vi "FTW-CodeGen-SelectMenu5.vi"(0 "State In":T2 {"Width" format="%dpx"}, 5 "XRef":refnum<vi>, 7 "Tag":string, 9 "Point":cluster{"H":i32, "V":i32}, 11 "Menu Type":T3(ring)) -> (4 "State Out":T2 {"Width" format="%dpx"}, 6 "Handled?":bool, 8 "Multi Object Popup Options":T1, 10 "Reply":string[](array[string]))   [LabVIEW 2015, in "FTW-Dataflow-Burrow.xnode"]
uses:
  FTW-Dataflow-Burrow.xnode
  FTW-CodeGen-State.ctl
  framework/FTW-CodeGen-XNodeReplyType.ctl
panel:
  # "Inputs"
  # "Outputs"
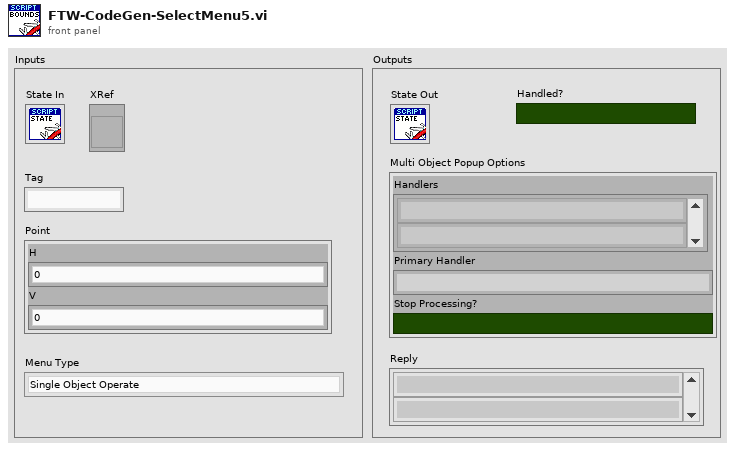
[diagram p1: front panel]
types:
  T1 = cluster{"Handlers":string[], "Primary Handler":string, "Stop Processing?":bool}
  T2 = typedef "FTW-Dataflow-Burrow.xnode/FTW-CodeGen-State.ctl" = cluster{"InputTerminals":cluster{"Wired?":bool, "ID":string, "DataName":string, "DataColor":u32, "Type":variant}[], "EnableTiming?":bool, "Width":i32}
  T3 = enum32{"Single Object Operate", "Single Object Popup", "Multi Object Popup Master", "Multi Object Popup Other"}
  T4 = typedef "FTW-CodeGen-XNodeReplyType.ctl" = enum16{"NoReply", "ForceAdaptToInputs", "UpdateTerms", "GenCode", "GenCode+CosmeticUpdate"}
  T5 = cluster{"Wired?":bool, "ID":string, "DataName":string, "DataColor":u32, "Type":variant}[]
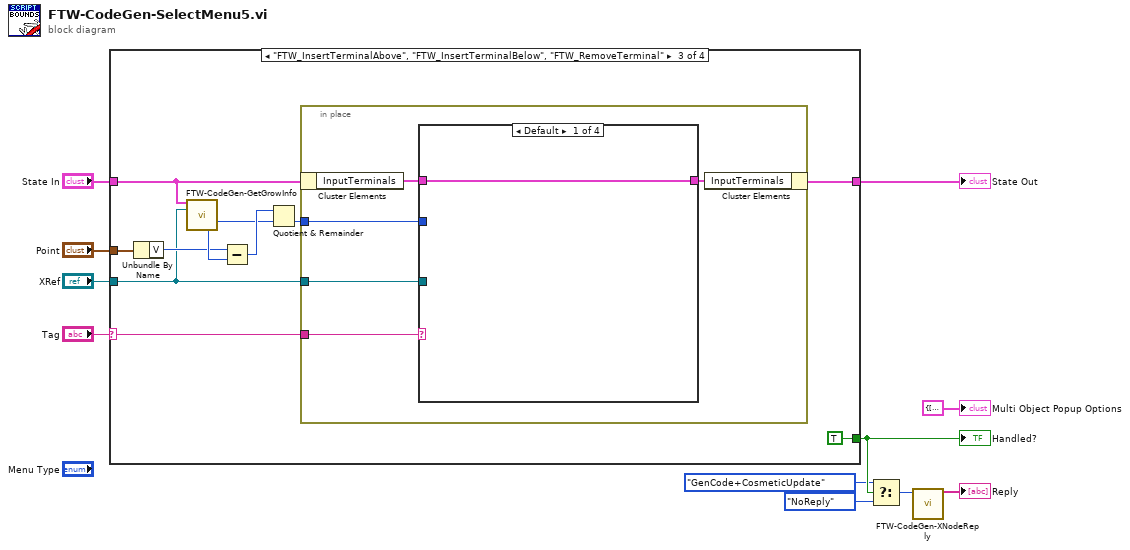
[diagram p0: block diagram]
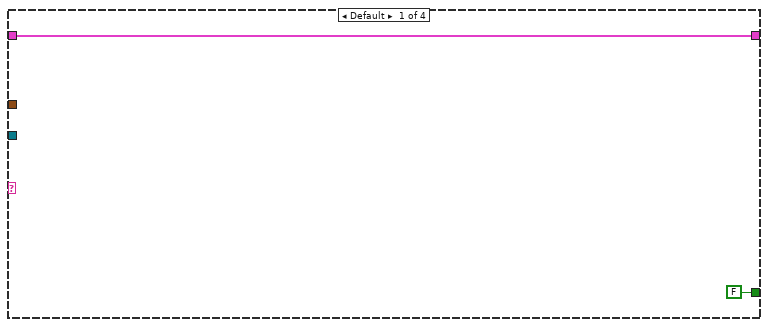
[diagram p2: hidden frame]
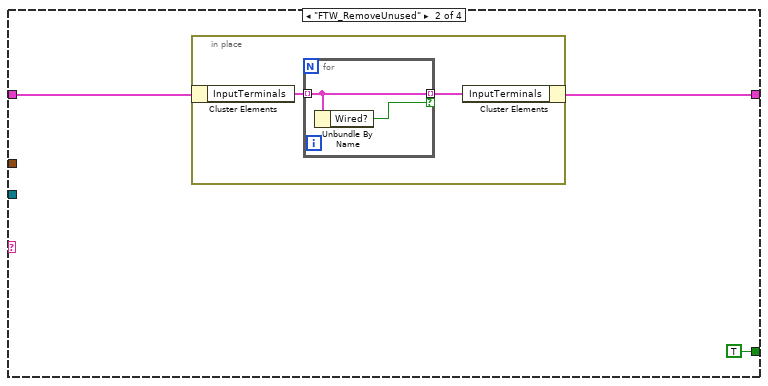
[diagram p3: hidden frame]
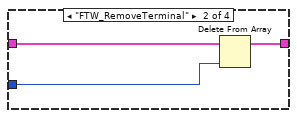
[diagram p4: hidden frame]
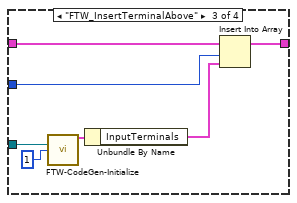
[diagram p5: hidden frame]
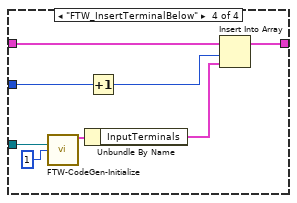
[diagram p6: hidden frame]
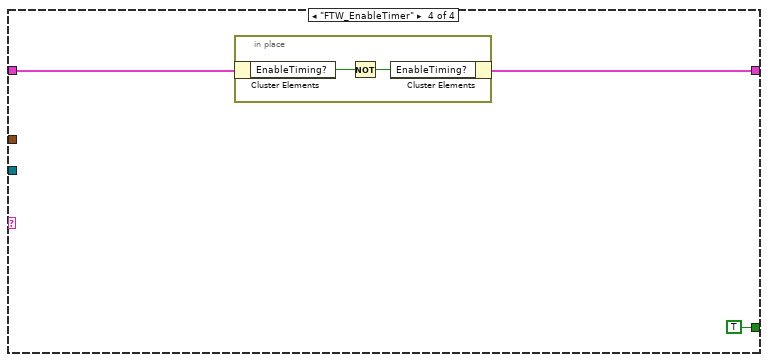
[diagram p7: hidden frame]
diagram:
  n1 = case shown="\"FTW_InsertTerminalAbove\", \"FTW_InsertTerminalBelow\", \"FTW_RemoveTerminal\"" "Tag" {
    selector: "Tag" -> [_ _ w22 _]
    tunnel: "XRef" -> [_ _ w21 _]
    tunnel: "State In" -> [w13 w16 w25 w57]
    tunnel: "Point" -> [_ _ w28 _]
    tunnel: [w13 w15 w24 w56] -> w2
    tunnel: [FALSE ("Handled?") TRUE ("Handled?") TRUE ("Handled?") TRUE ("Handled?")] -> w4
    frame Default {
    }
    frame "FTW_RemoveUnused" {
      n2 = in-place {
        n3 = in-place-cluster #1(w16) -> ("InputTerminals"=w18:T5)
        n4 = for {
          tunnel: w18 -> [w20] mode=indexing
          tunnel: [w20] -> w17 mode=indexing if=w19
          n5 = Unbundle By Name(w20) -> ("Wired?"=w19:bool)
        }
        n6 = in-place-cluster #1("InputTerminals"=w17) -> (w15:T2)
      }
    }
    frame "FTW_InsertTerminalAbove", "FTW_InsertTerminalBelow", "FTW_RemoveTerminal" {
      n7 = Unbundle By Name(w28) -> ("V"=w27:i32)
      n8 = call "FTW-CodeGen-GetGrowInfo.vi"("State In"=w25, "XRef"=w21) -> ("Terminal Height"=w29:i32, "Total Top Banner Height"=w31:i32)  [unwired: 5 in, 7 out]
      n9 = Subtract(x=w27, y=w31) -> (x-y=w30:i32)
      n10 = Quotient & Remainder(x=w30, y=w29) -> (floor(x/y)=w23:i32)  [unwired: 1 out]
      n11 = in-place {
        in-place-border: w23 -> [w32]
        in-place-border: w22 -> [w34]
        in-place-border: w21 -> [w33]
        n12 = in-place-cluster #2(w25) -> ("InputTerminals"=w36:T5)
        n13 = case shown="Default" w34 {
          tunnel: w36 -> [w37 w40 w46 w54]
          tunnel: [w37 w39 w45 w53] -> w35
          tunnel: w33 -> [_ _ w44 w52]
          tunnel: w32 -> [_ w38 w42 w50]
          frame Default {
          }
          frame "FTW_RemoveTerminal" {
            n14 = Delete From Array(array=w40, index=w38) -> (array with subset deleted=w39:T5)  [unwired: 1 in, 1 out]
          }
          frame "FTW_InsertTerminalAbove" {
            n15 = call "FTW-CodeGen-Initialize.vi"("XRef"=w44, "Items"=1) -> ("State Out"=w47:T2)  [unwired: 13 in]
            n16 = Unbundle By Name(w47) -> ("InputTerminals"=w41:T5)
            n17 = Insert Into Array(array=w46, index=w42, new element=w41) -> (w45:T5)
          }
          frame "FTW_InsertTerminalBelow" {
            n18 = call "FTW-CodeGen-Initialize.vi"("XRef"=w52, "Items"=1) -> ("State Out"=w55:T2)  [unwired: 13 in]
            n19 = Unbundle By Name(w55) -> ("InputTerminals"=w49:T5)
            n20 = Increment(x=w50) -> (x+1=w48:i32)
            n21 = Insert Into Array(array=w54, index=w48, new element=w49) -> (w53:T5)
          }
        }
        n22 = in-place-cluster #2("InputTerminals"=w35) -> (w24:T2)
      }
    }
    frame "FTW_EnableTimer" {
      n23 = in-place {
        n24 = in-place-cluster #3(w57) -> ("EnableTiming?"=w60:bool)
        n25 = Not(x=w60) -> (.not. x?=w59:bool)
        n26 = in-place-cluster #3("EnableTiming?"=w59) -> (w56:T2)
      }
    }
  }
  "State Out" <- w2
  "Handled?" <- w4
  n27 = Select(t=FTW-CodeGen-XNodeReplyType."GenCode+CosmeticUpdate", s=w4, f=FTW-CodeGen-XNodeReplyType."NoReply" ("XNode Reply Type")) -> (s? t:f=w3:T4)
  n28 = call "FTW-CodeGen-XNodeReply.vi"("XNode Reply Type"=w3) -> ("Reply"=→"Reply":string[])  [unwired: 14 in]
  "Multi Object Popup Options" <- T1 {"Handlers"=[], "Primary Handler"="", "Stop Processing?"=FALSE} ("Multi Object Popup Options")
